vi "test - Round Trip - Numeric - U8.vi"(8 "error in (no error)":errorcluster, 11 "TestCase in":refnum<class "Python Data Tools Tests.lvclass">) -> (0 "error out":errorcluster, 3 "TestCase out":refnum<class "Python Data Tools Tests.lvclass">)   [LabVIEW 2013, in "Python Data Tools Tests.lvclass"]
uses:
  Python Data Tools Tests.lvclass
  <vilib>/addons/_JKI Toolkits/VI Tester/TestCase.llb/TestCase.lvclass
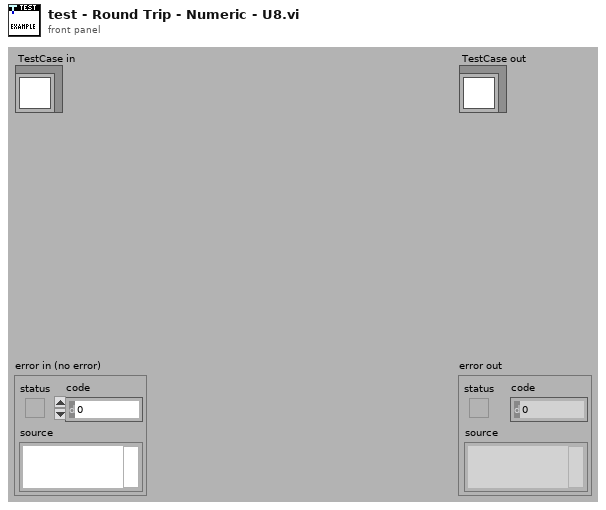
[diagram p1: front panel]
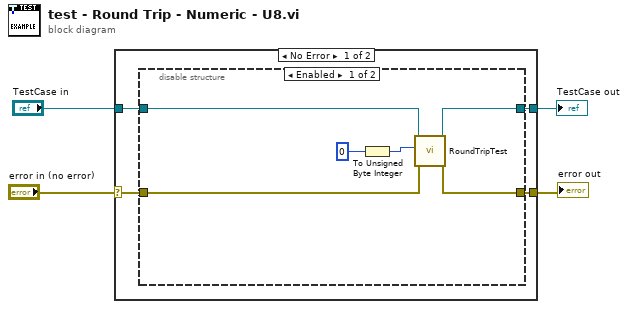
[diagram p0: block diagram]
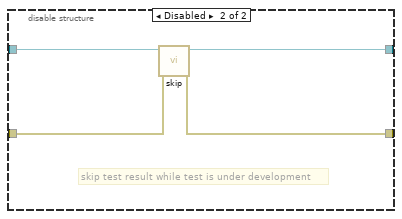
[diagram p2: hidden frame]
diagram:
  n1 = case shown="No Error" "error in (no error)" {
    selector: "error in (no error)" -> [w6 w20]
    tunnel: [w5 w20] -> w3
    tunnel: [w7 w19] -> w1
    tunnel: "TestCase in" -> [w8 w19]
    frame No Error {
      n2 = disable-structure shown="Enabled" {
        disable-tunnel: w8 -> [w14 w18]
        disable-tunnel: [w13 w15] -> w7
        disable-tunnel: w6 -> [w11 w17]
        disable-tunnel: [w12 w16] -> w5
        frame Enabled {
          n3 = To Unsigned Byte Integer(number=u8 0) -> (unsigned 8bit integer=w9:u8)
          n4 = call "RoundTripTest.vi"("error in (no error)"=w11, "Variant"=w9, "TestCase in"=w14) -> ("error out"=w12:errorcluster, "TestCase out"=w13:refnum<class "Python Data Tools Tests.lvclass">)  [unwired: 6 in, 1 out]
        }
        frame Disabled {
          # "skip test result while test is under development"
          n5 = call <vilib>:"skip.vi"("error in (no error)"=w17, "TestCase in"=w18) -> ("error out"=w16:errorcluster, "TestCase out"=w15:refnum<class "Python Data Tools Tests.lvclass">)  [unwired: 8 in]
        }
      }
    }
    frame Error {
    }
  }
  "error out" <- w3
  "TestCase out" <- w1
